vi "SeqMgr.Initialize Seq, Init Return Info.vi"(8 "error in (no error)":errorcluster, 10 "Rtn Info":variant, 11 "SeqMgr in":refnum<class "SeqMgr.lvclass">) -> (0 "error out":errorcluster, 3 "SeqMgr out":refnum<class "SeqMgr.lvclass">)   [LabVIEW 2024, in "EQMF.lvlib" / "SeqMgr.lvlib" / "SeqMgr.lvclass"]
uses:
  SeqMgr.lvclass
  Queues/Q.Msg Return Info.ctl
  Queues/Q.Element.ctl
  SeqMgr.lvclass/SeqMgr.ctl
  Queues/Queue Utils.lvlib
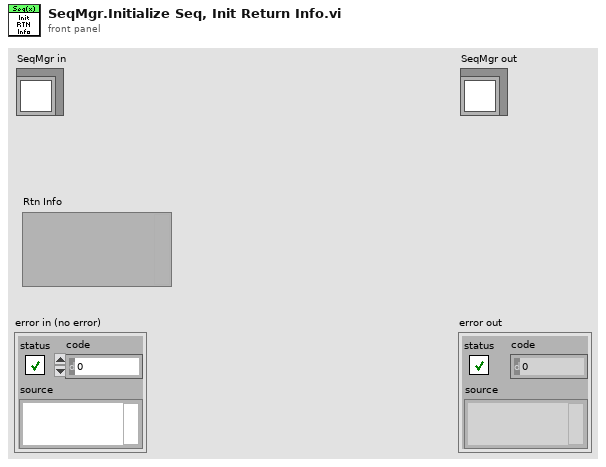
[diagram p1: front panel]
types:
  T1 = typedef "EQMF.lvlib/Queue Utils.lvlib/Q.Msg Return Info.ctl" = cluster{"Ret Q":refnum<queue>, "Ret Msg":T2, "SeqNum":i32}
  T2 = typedef "EQMF.lvlib/Queue Utils.lvlib/Q.Element.ctl" = cluster{"Cmd":string, "Sub":string, "Data1":variant, "Data2":variant}
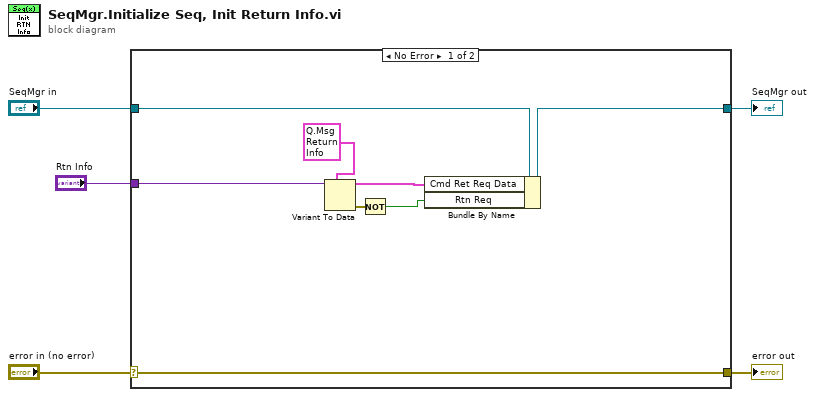
[diagram p0: block diagram]
diagram:
  n1 = case shown="No Error" "error in (no error)" {
    selector: "error in (no error)" -> [w13 w15]
    tunnel: [w13 w15] -> w4
    tunnel: [w11 w14] -> w2
    tunnel: "SeqMgr in" -> [w12 w14]
    tunnel: "Rtn Info" -> [w8 _]
    frame No Error {
      n2 = Variant To Data(type=T1 {"Ret Q"=refnum, "Ret Msg"={"Cmd"="", "Sub"="", "Data1"=variant, "Data2"=variant}, "SeqNum"=0} ("Cmd Ret Req Data"), Variant=w8) -> (data=w9:T1, error out=w7:errorcluster)  [unwired: 1 in]
      n3 = Not(x=w7) -> (.not. x?=w6:bool)
      n4 = Bundle By Name(cluster=w12, "Cmd Ret Req Data"=w9, "Rtn Req"=w6) -> (w11:refnum<class "SeqMgr.lvclass">)
    }
    frame Error {
    }
  }
  "error out" <- w4
  "SeqMgr out" <- w2
